vi "Test Settings Database.vi"(8 "error in (no error)":errorcluster) -> (0 "error out":errorcluster)   [LabVIEW 2019]
uses:
  <vilib>/addons/_JKI Toolkits/Caraya/classes/Test/Test.lvclass
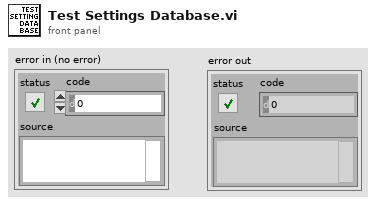
[diagram p1: front panel]
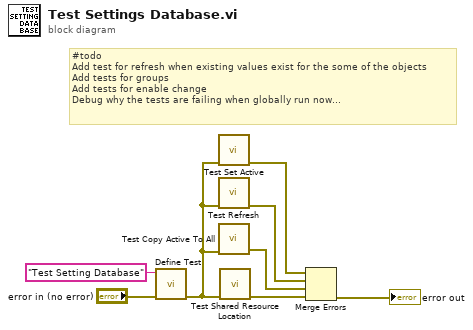
[diagram p0: block diagram]
diagram:
  # "#todo\nAdd test for refresh when existing values exist for the some of the objects\nAdd tests for groups\nAdd tests for enable change \nDebug why the tests are failing when globally run now..."
  n1 = call <vilib>:"Define Test.vi"("error in (no error)"="error in (no error)", "Label (VI Title)"="Test Setting Database") -> ("error out"=w1:errorcluster)  [unwired: 8 in, 1 out]
  n2 = call "Test Set Active.vi"("error in (no error)"=w1) -> ("error out"=w2:errorcluster)  [unwired: 10 in]
  n3 = call "Test Refresh.vi"("error in (no error)"=w1) -> ("error out"=w3:errorcluster)  [unwired: 10 in]
  n4 = call "Test Copy Active To All.vi"("error in (no error)"=w1) -> ("error out"=w4:errorcluster)  [unwired: 10 in]
  n5 = call "Test Shared Resource Location.vi"("error in"=w1) -> ("error out"=w6:errorcluster)  [unwired: 10 in]
  n6 = Merge Errors(w2, w3, w4, w6) -> (→"error out":errorcluster)
